vi "licdf device count.vi"(8 "error in (no error)":errorcluster, 11 "out_count":i32) -> (0 "error out":errorcluster, 2 "function return":i32, 3 "out_count out":i32)   [LabVIEW 2026, in "keynub_licdongle.lvlib"]
doc: "int32_t licdf_device_count(int32_t *out_count);"
uses:
  keynub_licdongle.lvlib
  natives/win-x64/keynub_licdongle_flat.dll
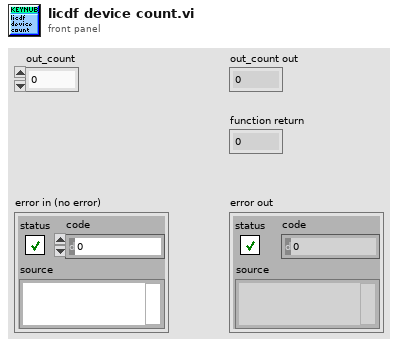
[diagram p1: front panel]
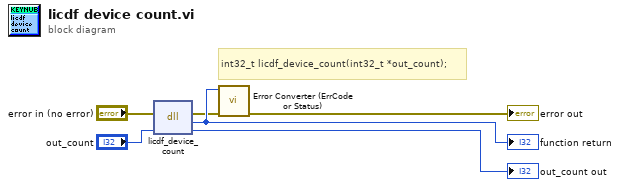
[diagram p0: block diagram]
diagram:
  # "int32_t licdf_device_count(int32_t *out_count);"
  n1 = dll-call lib="C:/Austausch/KeyNub/LicenseDongle-PublicSDK/natives/win-x64/keynub_licdongle_flat.*" fn="licdf_device_count"(error in="error in (no error)", "out_count"="out_count") -> (error out=w2:errorcluster, w6:i32, "out_count"=→"out_count out":i32)  [unwired: 2 in, 1 out]
  "function return" <- w6
  n2 = call "Error Converter (ErrCode or Status).vi"("error in (no error)"=w2, "error code"=w6) -> ("error out"=→"error out":errorcluster)  [unwired: 9 in]
